vi "Remove Assert VIs From Call Chain.vi"(11 "call chain in":string[](array[string])) -> (3 "call chain out":string[](array[string]))   [LabVIEW 2013, in "Caraya.lvlib" / "Assert.lvclass"]
doc: "Given a call chain, drop the front part of the array up to and including the last item that is found in the <b>Registry For Assert VIs</b>. This leaves a call chain that starts with a VI that is in the caller's actual test suite where <b>Define Test</b> is expected to be called."
uses:
  Assert.lvclass
  Registry For Assert VIs.vi
  <vilib>/regexp/Match Regular Expression.xnode
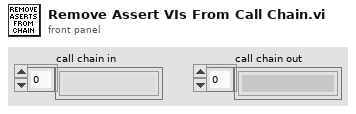
[diagram p1: front panel]
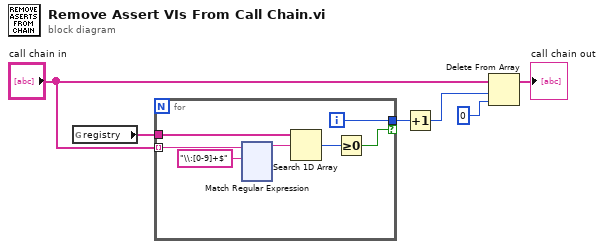
[diagram p0: block diagram]
diagram:
  n1 = global read "Registry For Assert VIs.vi" "registry"() -> (w4:string[])
  n2 = for {
    tunnel: "call chain in" -> [w8] mode=indexing
    tunnel: w4 -> [w13]
    tunnel: [w12] -> w2 if=w10
    i -> [w12]
    n3 = xnode "Match Regular Expression"("input string"=w8, "regular expression"="\\:[0-9]+$") -> ("before match"=w7:string)  [unwired: 4 in, 4 out]
    n4 = Search 1D Array(1D array=w13, element=w7) -> (index of element=w11:i32)  [unwired: 1 in]
    n5 = Greater Or Equal To 0?(x=w11) -> (x >= 0?=w10:bool)
  }
  n6 = Increment(x=w2) -> (x+1=w1:i32)
  n7 = Delete From Array(array="call chain in", length=w1, index=0) -> (array with subset deleted=→"call chain out":string[])  [unwired: 1 out]
